vi "VI Tree - xxx- Files.vi"   [LabVIEW 2020]
uses:
  openg_array.lvlib
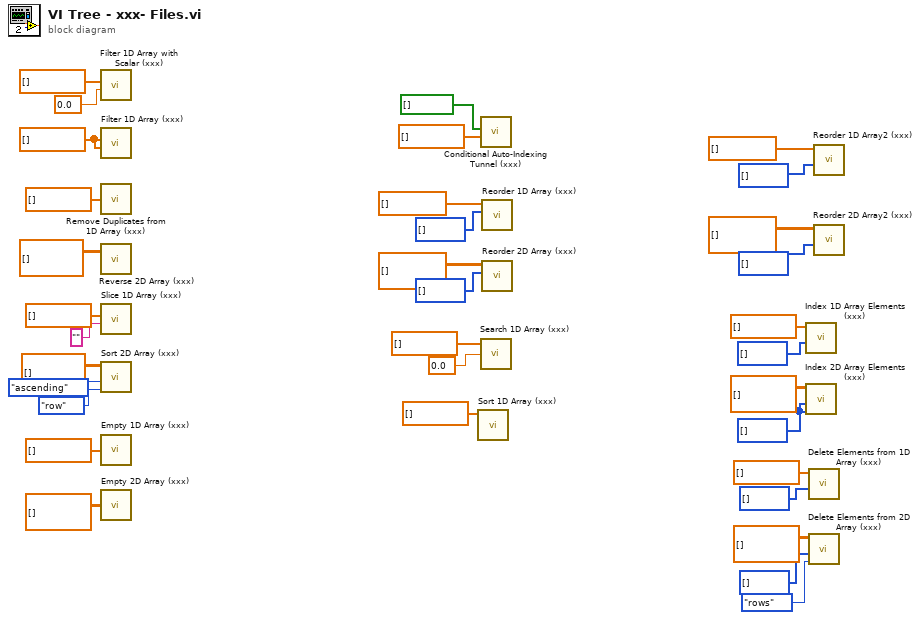
[diagram p0: block diagram]
diagram:
  w1 = i32[] [] ("indices")
  w33 = dbl[] [] ("Array")
  n1 = call "Filter 1D Array with Scalar (xxx).vi"("items to filter"=0.0 ("Numeric"), "array"=dbl[] [] ("Array")) -> ()  [unwired: 4 in, 2 out]
  n2 = call "Filter 1D Array (xxx).vi"("items to filter"=w33, "array"=w33) -> ()  [unwired: 4 in, 2 out]
  n3 = call "Remove Duplicates from 1D Array (xxx).vi"("Input Array"=dbl[] []) -> ()  [unwired: 2 out]
  n4 = call "Reverse 2D Array (xxx).vi"("Array"=dbl[][] []) -> ()  [unwired: 2 in, 1 out]
  n5 = call "Slice 1D Array (xxx).vi"("slice"="", "array"=dbl[] []) -> ()  [unwired: 5 in, 1 out]
  n6 = call "Sort 2D Array (xxx).vi"("Sort By in"=enum16{"row", "column"}."row", "Order"=enum16{"ascending", "descending"}."ascending", "Array in"=dbl[][] []) -> ()  [unwired: 5 in, 4 out]
  n7 = call "Empty 1D Array (xxx).vi"("Array"=dbl[] []) -> ()  [unwired: 8 in, 1 out]
  n8 = call "Empty 2D Array (xxx).vi"("Array"=dbl[][] []) -> ()  [unwired: 8 in, 1 out]
  n9 = call "Sort 1D Array (xxx).vi"("Array in"=dbl[] []) -> ()  [unwired: 9 in, 2 out]
  n10 = call "Conditional Auto-Indexing Tunnel (xxx).vi"("Array in"=dbl[] [], "Elements to keep"=bool[] []) -> ()  [unwired: 5 in, 1 out]
  n11 = call "Search 1D Array (xxx).vi"("Array"=dbl[] [], "Element Data"=0.0) -> ()  [unwired: 7 in, 1 out]
  n12 = call "Reorder 1D Array (xxx).vi"("Sorted Pointers in"=i32[] [], "Array in"=dbl[] []) -> ()  [unwired: 8 in, 2 out]
  n13 = call "Reorder 2D Array (xxx).vi"("Sorted Pointers in"=i32[] [], "Array in"=dbl[][] []) -> ()  [unwired: 7 in, 3 out]
  n14 = call "Index 1D Array Elements (xxx).vi"("indices"=i32[] [], "array"=dbl[] []) -> ()  [unwired: 9 in, 1 out]
  n15 = call "Index 2D Array Elements (xxx).vi"("indices 1"=w1, "indices 0"=w1, "array"=dbl[][] []) -> ()  [unwired: 8 in, 1 out]
  n16 = call "Delete Elements from 1D Array (xxx).vi"("indices"=i32[] [], "array"=dbl[] []) -> ()  [unwired: 8 in, 2 out]
  n17 = call "Delete Elements from 2D Array (xxx).vi"("delete (rows or columns)"=enum16{"rows", "columns"}."rows", "indices"=i32[] [], "array"=dbl[][] []) -> ()  [unwired: 7 in, 2 out]
  n18 = call "Reorder 1D Array2 (xxx).vi"("indices"=i32[] [] ("Sorted Pointers in"), "array"=dbl[] [] ("Array in")) -> ()  [unwired: 9 in, 1 out]
  n19 = call "Reorder 2D Array2 (xxx).vi"("indices"=i32[] [] ("Sorted Pointers in"), "array"=dbl[][] [] ("Array in")) -> ()  [unwired: 9 in, 1 out]
